vi "Pseudo Heart Rate Indicators.vi"() -> ()   [LabVIEW 2013]
panel:
  out "Normal":bool
  in  "stop":bool
  out "Bradycardia":bool
  out "Tachycardia":bool
  out "Crude Heart Rate Monitor":dbl(slide) scale=0.0..150.0
  in  "Crude Heart Rate":dbl(slide) scale=0.0..150.0
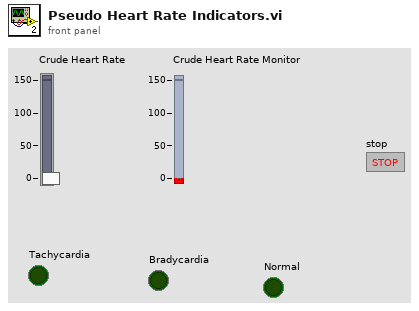
[diagram p1: front panel]
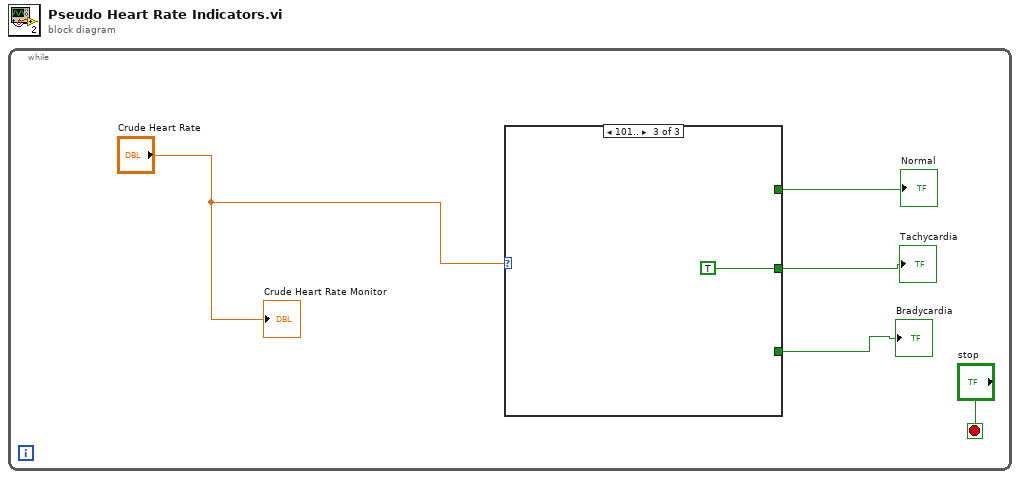
[diagram p0: block diagram]
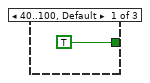
[diagram p2: hidden frame]
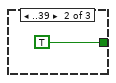
[diagram p3: hidden frame]
diagram:
  n1 = while {
    stop <- "stop" stop-if-true
    n2 = case shown="101.." "Crude Heart Rate" {
      tunnel: [TRUE _ _] -> w3
      tunnel: [_ TRUE _] -> w2
      tunnel: [_ _ TRUE] -> w1
      frame 40..100, Default {
      }
      frame ..39 {
      }
      frame 101.. {
      }
    }
    "Tachycardia" <- w1
    "Bradycardia" <- w2
    "Normal" <- w3
    "Crude Heart Rate Monitor" <- "Crude Heart Rate"
  }
